vi "merge_Timer On Delay.vi"   [LabVIEW 2020, in "NI_FunctionBlockMergeVIs.lvlib"]
doc: "Generates an <B>output</B> signal with falling edges that align with those of the <B>input</B> signal, but with rising edges delayed by <B>preset time (ms)</B>."
uses:
  <vilib>/functionblocks/NI_FunctionBlockMergeVIs.lvlib
  <vilib>/functionblocks/FB Core/FB Core.xnode
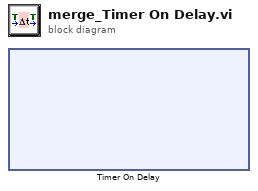
[diagram p0: block diagram]
diagram:
  n1 = xnode "Timer On Delay"() -> ()  [unwired: 3 in, 3 out]
